vi "Phasor Is (g,s) on UC.vi"(2 "Phasor (g, s)":T1) -> (7 "Is on UC?":bool)   [LabVIEW 2021, in "Phasor.lvlib"]
doc: "Verifies that g^2+ s^2 = g, which is the definition of the universal circle."
uses:
  Phasor.lvlib
  Phasor (g, s).ctl
  08b24e8a-c6d5-4f8d-ba09-80eb33e27d4b.vi
  08b24e8a-c6d5-4f8d-ba09-80eb33e27d4b.vi/8a80743f-1319-44c8-96b0-3ef8fc688731.vi
  08b24e8a-c6d5-4f8d-ba09-80eb33e27d4b.vi/931f4f8f-d8c6-4056-833f-5c8fe97b24b9.vi
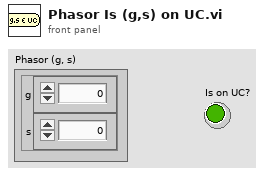
[diagram p1: front panel]
types:
  T1 = typedef "Phasor.lvlib/Phasor (g, s).ctl" = cluster{"g":dbl, "s":dbl}
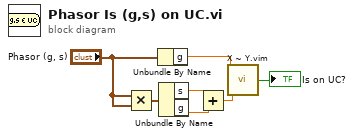
[diagram p0: block diagram]
diagram:
  n1 = Multiply(x="Phasor (g, s)", y="Phasor (g, s)") -> (x*y=w6:T1)
  n2 = Unbundle By Name("Phasor (g, s)") -> ("g"=w2:dbl)
  n3 = Unbundle By Name(w6) -> ("s"=w5:dbl, "g"=w4:dbl)
  n4 = Add(x=w5, y=w4) -> (x+y=w3:dbl)
  n5 = call "X ~ Y.vim"("X"=w2, "Y"=w3) -> ("X ~= Y?"=→"Is on UC?":bool)  [unwired: 13 in]
